vi "PI_valvula7.vi"(9 "controlON":bool, 10 "Temperatura":dbl format="%.2f", 11 "Setpoint T":dbl) -> (3 "PWM (%)":dbl)   [LabVIEW 2022 SP3, in "DAQ_Termopares.lvlib"]
uses:
  DAQ/DAQ_Termopares.lvlib
  <vilib>/addons/control/pid/pid.llb/PID (DBL).vi
  <vilib>/addons/control/pid/NI_PID_pid.lvlib
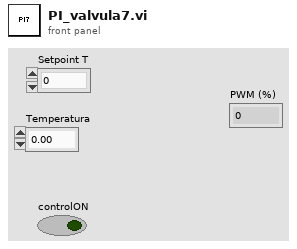
[diagram p1: front panel]
types:
  T1 = cluster{"proportional gain (Kc)":dbl, "integral time (Ti, min)":dbl, "derivative time (Td, min)":dbl}
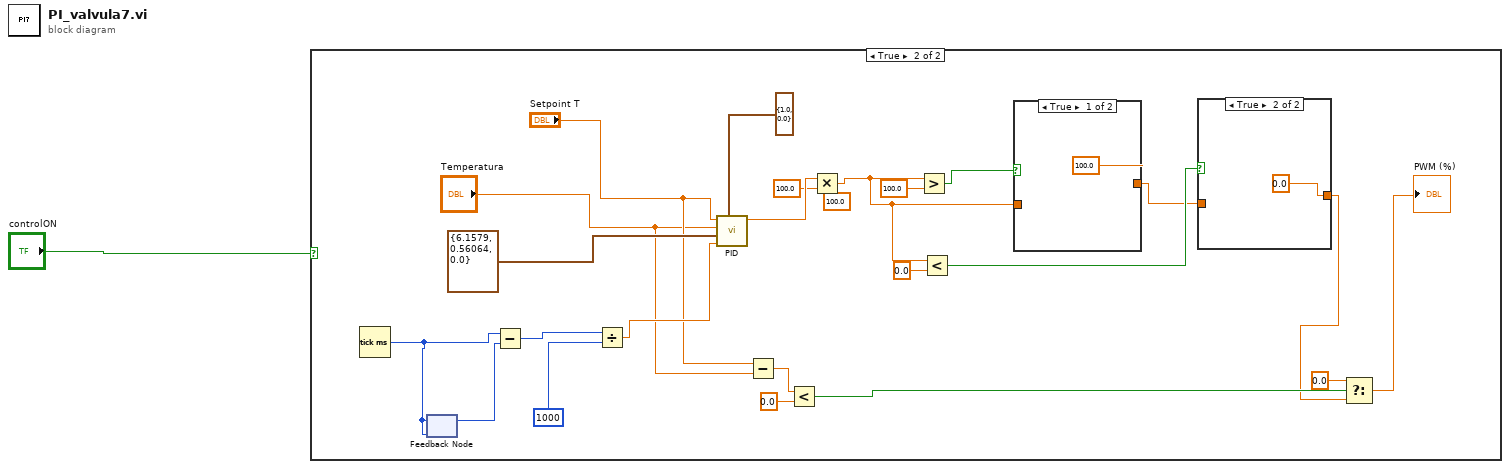
[diagram p0: block diagram]
diagram:
  n1 = case shown="True" "controlON" {
    frame False {
    }
    frame True {
      (unwired) 100.0 ("y")
      n2 = Tick Count (ms)() -> (millisecond timer value=w24:u32)
      n3 = feedback #1(w24) -> (w23:u32)
      n4 = feedback-in #1(w24) -> ()
      n5 = Subtract(x=w24, y=w23) -> (x-y=w21:u32)
      n6 = Divide(x=w21, y=1000) -> (x/y=w10:dbl)
      n7 = call-poly <vilib>:"PID.vi"("output range"=cluster{"output high":dbl, "output low":dbl} {"output high"=1.0, "output low"=0.0}, "dt (s)"=w10, "PID gains"=T1 {"proportional gain (Kc)"=6.1579, "integral time (Ti, min)"=0.56064, "derivative time (Td, min)"=0.0}, "process variable"="Temperatura", "setpoint"="Setpoint T") -> ("output"=w18:dbl)  [unwired: 5 in, 1 out]
      n8 = Subtract(x="Setpoint T", y="Temperatura") -> (x-y=w9:dbl)
      n9 = Less?(x=w9, y=0.0) -> (x < y?=w7:bool)
      n10 = Multiply(x=w18, y=100.0) -> (x*y=w13:dbl)
      n11 = Greater?(x=w13, y=100.0) -> (0:w14:bool)
      n12 = Less?(x=w13, y=0.0) -> (x < y?=w12:bool)
      n13 = case shown="True" w14 {
        tunnel: w13 -> [_ w28]
        tunnel: [100.0 w28] -> w11
        frame True {
        }
        frame False {
        }
      }
      n14 = case shown="True" w12 {
        tunnel: w11 -> [w25 _]
        tunnel: [w25 0.0] -> w3
        frame False {
        }
        frame True {
        }
      }
      n15 = Select(t=0.0, s=w7, f=w3) -> (s? t:f=→"PWM (%)":dbl)
    }
  }
